vi "Actor Core.vi"(8 "error in":errorcluster, 11 "Actor in":refnum<class "Actor.lvclass">) -> (0 "error out":errorcluster, 3 "Actor out":refnum<class "Actor.lvclass">)   [LabVIEW 2020, in "Actor Framework.lvlib" / "Actor.lvclass"]
doc: "(<B>Filename</B>: Actor Framework.lvlib:Actor.lvclass:Actor Core.vi)\n\nReceives messages to the actor, reacts to them, and initiates any error handling that may shut the actor down.\n\nDescendant classes may override this VI to append parallel tasks for the actor to complete while it handles messages. Overrides use the Call Parent Class Method node."
uses:
  <vilib>/ActorFramework/Actor/Actor.lvclass
  <vilib>/ActorFramework/Actor/Actor.lvclass/Actor.ctl
  <vilib>/ActorFramework/Message Priority Queue/Message Priority Queue.lvclass
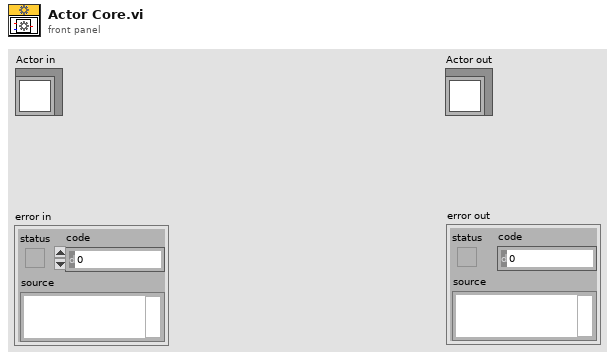
[diagram p1: front panel]
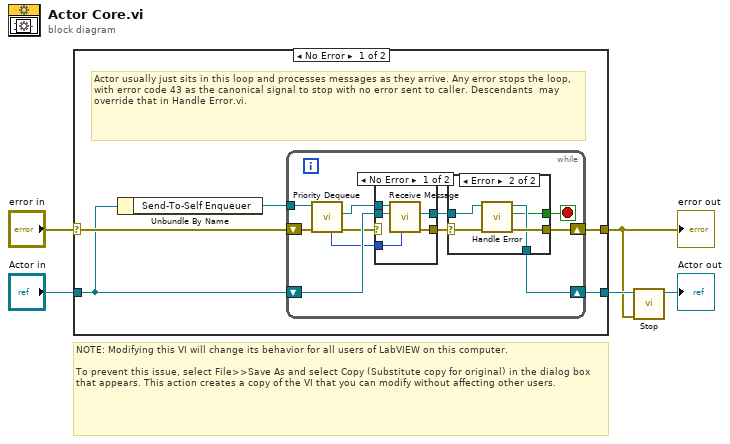
[diagram p0: block diagram]
diagram:
  # "NOTE: Modifying this VI will change its behavior for all users of LabVIEW on this computer.\n\nTo prevent this issue, select File>>Save As and select Copy (Substitute copy for original) in the dialog box that appears. This action creates a copy of the VI that you can modify without affecting other users."
  n1 = case shown="No Error" "error in" {
    selector: "error in" -> [w10 w37]
    tunnel: [w8 w37] -> w1
    tunnel: "Actor in" -> [w6 w36]
    tunnel: [w7 w36] -> w3
    frame No Error {
      # "Actor usually just sits in this loop and processes messages as they arrive. Any error stops the loop, with error code 43 as the canonical signal to stop with no error sent to caller. Descendants  may override that in Handle Error.vi."
      n2 = Unbundle By Name(w6) -> ("Send-To-Self Enqueuer"=w9:refnum<class "Message Priority Queue.lvclass">)
      n3 = while {
        tunnel: w9 -> [w16]
        shift-right: [w18] -> w7
        shift-left: w6 -> [w21]
        shift-right: [w19] -> w8
        shift-left: w10 -> [w20]
        stop <- w14 stop-if-true
        n4 = call <vilib>:"Priority Dequeue.vi"("error in (no error)"=w20, "Priority Queue in"=w16) -> ("error out"=w11:errorcluster, "element"=w17:refnum<class "Message.lvclass">, "priority"=w12:i32)  [unwired: 5 in, 2 out]
        n5 = case shown="No Error" w11 {
          selector: w11 -> [_ w27]
          tunnel: w21 -> [w26 w28]
          tunnel: w17 -> [w25 _]
          tunnel: [w24 w27] -> w15
          tunnel: [w23 w28] -> w13
          tunnel: w12 -> [w22 _]
          frame No Error {
            n6 = call-dynamic "Receive Message.vi"("priority"=w22, "Actor in"=w26, "Message in"=w25) -> ("error out"=w24:errorcluster, "Actor out"=w23:refnum<class "Actor.lvclass">)  [unwired: 7 in]
          }
          frame Error {
          }
        }
        n7 = case shown="Error" w15 {
          selector: w15 -> [w29 w32]
          tunnel: [w29 w35] -> w19
          tunnel: w13 -> [w30 w34]
          tunnel: [w30 w33] -> w18
          tunnel: [_ w31] -> w14
          frame No Error {
          }
          frame Error {
            n8 = call-dynamic "Handle Error.vi"("error in (no error)"=w32, "Actor in"=w34) -> ("error out"=w35:errorcluster, "stop actor?"=w31:bool, "Actor out"=w33:refnum<class "Actor.lvclass">)  [unwired: 7 in]
          }
        }
      }
    }
    frame Error {
    }
  }
  "error out" <- w1
  n9 = call <vilib>:"Stop.vi"("error in"=w1, "Actor in"=w3) -> ("Actor out"=→"Actor out":refnum<class "Actor.lvclass">)  [unwired: 9 in]
